vi "ProyectoBioCuinique Alpha 3.0.vi"() -> ()   [LabVIEW 2021]
uses:
  <vilib>/Utility/NIReport.llb/Report Type.ctl
  <extravilib>/ChannelInstances/Tag-dbl/Read With Abort.vi
  <extravilib>/ChannelInstances/Tag-bool/Read With Abort.vi
  <extravilib>/ChannelInstances/Tag-bool/Write With Abort.vi
  <extravilib>/ChannelInstances/Tag-dbl/Write With Abort.vi
  <vilib>/Instr/_visa.llb/VISA Configure Serial Port (Instr).vi
  <vilib>/MakerHub/LINX/Public/Utilities/Open Serial.vi
  <extravilib>/ChannelInstances/Tag-dbl/Instantiate.vi
  <extravilib>/ChannelInstances/Tag-bool/Instantiate.vi
  <extravilib>/ChannelInstances/Tag-dbl/EndpointRead.vi
  <vilib>/addons/_office/excel.llb/Excel Easy Table (str).vi
  <extravilib>/ChannelInstances/Tag-bool/EndpointRead.vi
  <extravilib>/ChannelInstances/Tag-bool/Endpoint.vi
  <extravilib>/ChannelInstances/Tag-dbl/Endpoint.vi
  <vilib>/Utility/NIReport.llb/NI_report.lvclass
  <vilib>/LabVIEW Interface for Arduino/LabVIEW Interface for Arduino.lvlib
  <vilib>/MakerHub/LINX/LMH-LINX.lvlib
  <vilib>/Utility/NIReport.llb/NI_ReportGenerationCore.lvlib
  <vilib>/addons/_office/NI_ReportGenerationToolkit.lvlib
  <vilib>/Utility/NIReport.llb/Excel/NI_Excel.lvclass
  <vilib>/MakerHub/LINX/Public/Sensors/Distance/Ultrasonic/Ultrasonic.lvlib
  <extravilib>/ChannelInstances/Tag-bool.lvlib
  <extravilib>/ChannelInstances/Tag-dbl.lvlib
panel:
  in  "Serial Port":refnum<visa-resource-name>="N/A"
  in  "template (empty)":path
  in  "Pin Bomba 1":u8
  in  "Pin Valvula 1":u8
  in  "Pin Valvula 2":u8
  out "HUMEDAD 2":dbl
  in  "VISA resource name":refnum<visa-resource-name>
  out "TEMPERATURA":dbl
  out "HUMEDAD":dbl(knob) scale=0.0..255.0
  out "Centimeters":dbl
  out "Slide":dbl(slide) scale=0.0..500.0
  out "BOMBA (11)":bool
  in  "Boolean 4":bool
  out "VALVULA (6)":bool
  in  "Boolean":bool
  out "VALVULA (5)":bool
  in  "stop":bool
  in  "VISA resource":refnum<visa-resource-name>
  # "VÁLVULA 1"
  # "BOMBA DE AGUA"
  # "VÁLVULA 2"
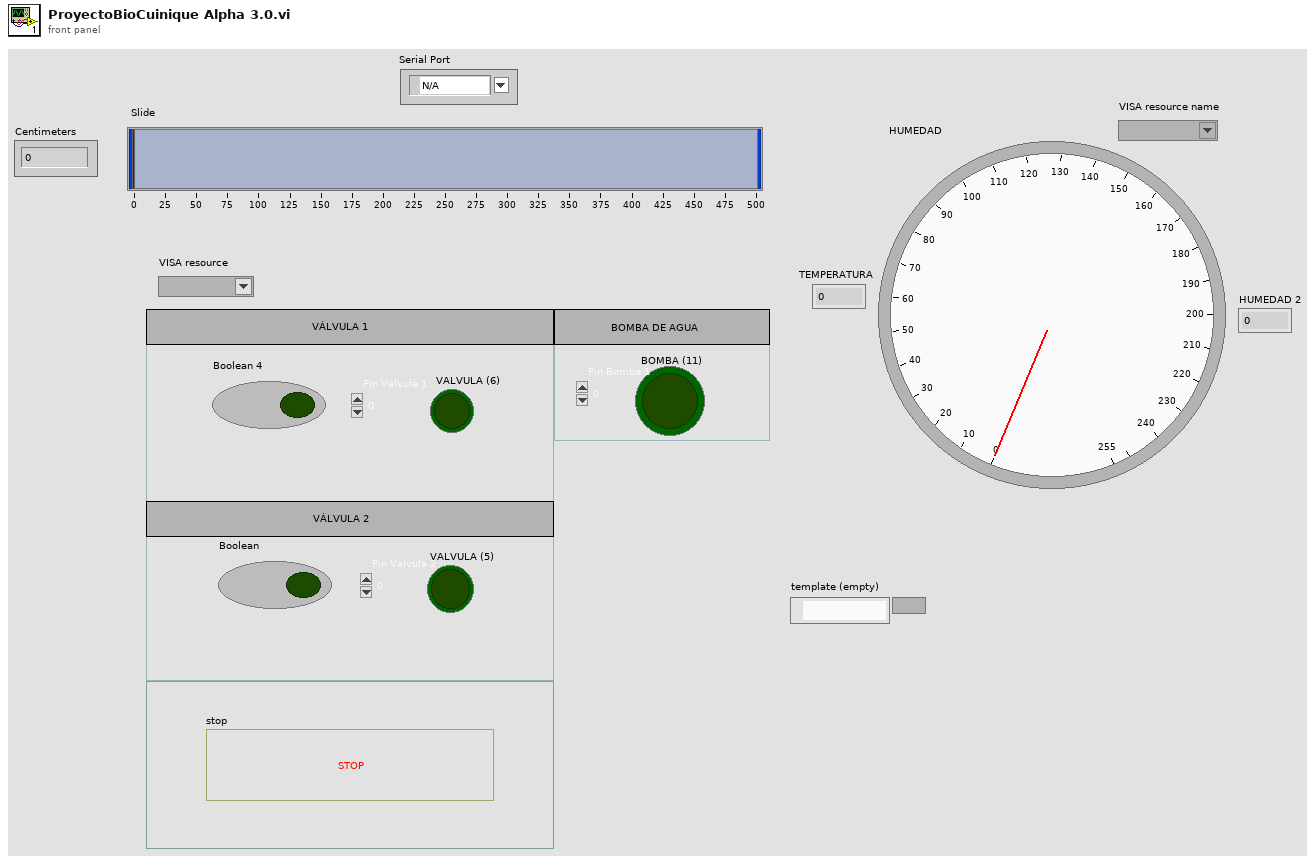
[diagram p1: front panel]
types:
  T1 = typedef "NI_ReportGenerationCore.lvlib/Report Type.ctl" = enum16{"HTML", "Word", "Excel"}
  T2 = typedef "LabVIEW Interface for Arduino.lvlib/Arduino Resource.ctl" = cluster{"VISA resource":refnum<visa-resource-name>, "Board Type":T3, "Connection Type":enum8{"USB / Serial"}, "Bytes Per Packet (15)":u8}
  T3 = typedef "LabVIEW Interface for Arduino.lvlib/Board Type.ctl" = enum16{"Uno", "Dimuelanove w/Atmega 328", "Mega 2560"}
  T4 = typedef "LMH-LINX.lvlib/LINX Ref.ctl" = cluster{"IO":T5, "Interface":T6, "LINX Device Config":T7}
  T5 = typedef "LMH-LINX.lvlib/Platform.ctl" = enum16{"Remote", "Local"}
  T6 = typedef "LMH-LINX.lvlib/Interface.ctl" = enum16{"Serial", "TCP"}
  T7 = typedef "LMH-LINX.lvlib/Device.lvlib/LINX Device Config.ctl" = cluster{"Interface":T6, "COM Port":refnum<visa-resource-name>, "TCP Configuration":T8, "Device Family":u8, "Device ID":u8, "Device Name":string, "TCP Ref":refnum<k5>, "Channels":T9}
  T8 = typedef "LMH-LINX.lvlib/Device.lvlib/TCP Config.ctl" = cluster{"IP Address":string, "Port":u16}
  T9 = typedef "LMH-LINX.lvlib/Channels.ctl" = cluster{"DI":u8[], "DO":u8[], "AI":u8[], "AO":u8[], "PWM":u8[], "QE":u8[], "UART":u8[], "I2C 2":u8[], "SPI":u8[], "CAN":u8[], "Servo":u8[], "AI Ref (V)":dbl, "AI Resolution (Bits)":u8, "AO Ref (V)":dbl, "AO Resolution (Bits)":u8}
  T10 = typedef "Tag-dbl.lvlib/))Channel.ctl" = refnum<queue>
  T11 = typedef "Tag-bool.lvlib/))Channel.ctl" = refnum<queue>
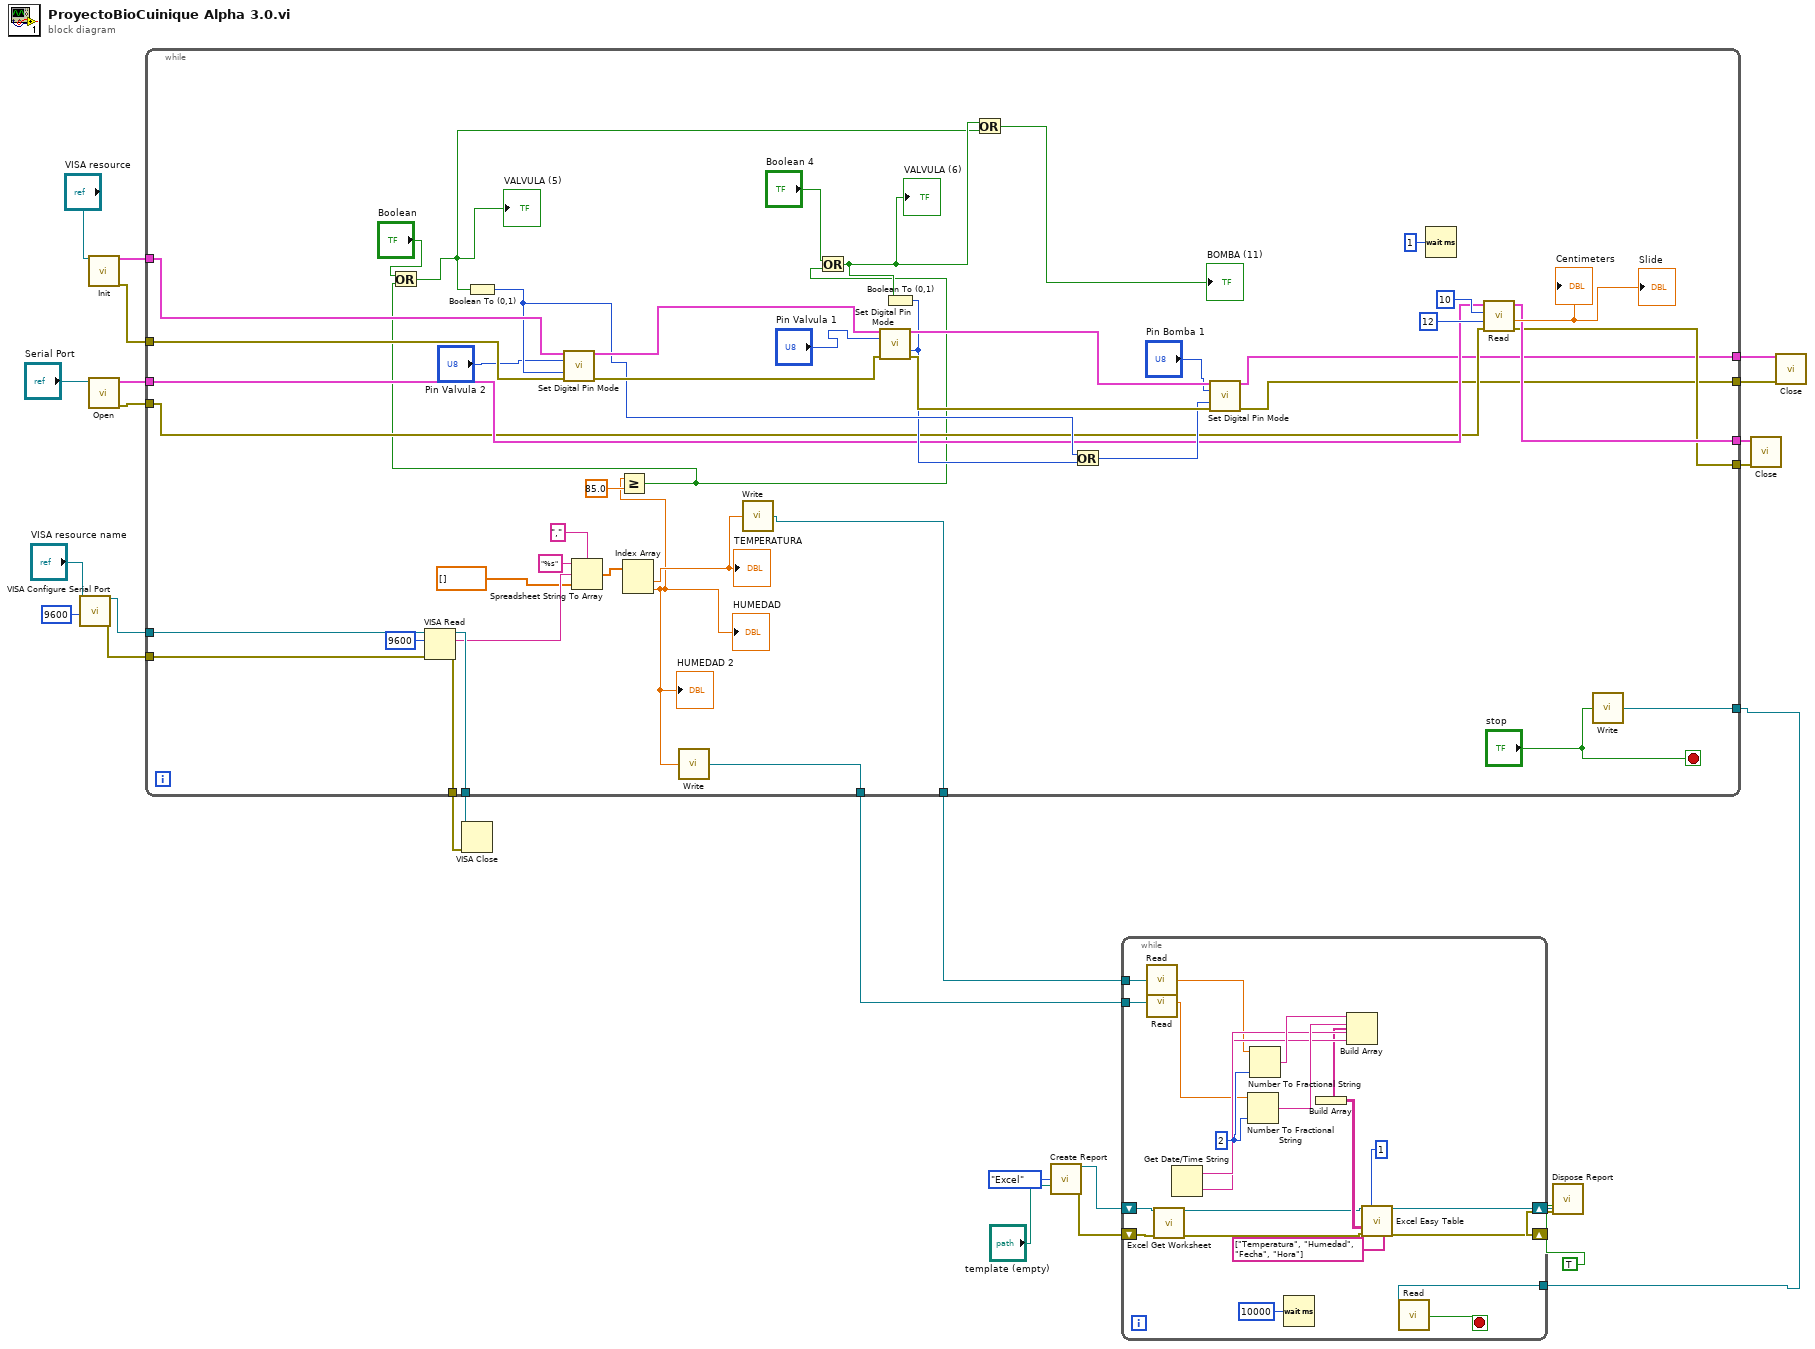
[diagram p0: block diagram]
diagram:
  n1 = call-poly "VISA Configure Serial Port"("VISA resource name"="VISA resource name", "baud rate (9600)"=u32 9600) -> ("VISA resource name out"=w17:refnum<visa-resource-name>, "error out"=w14:errorcluster)  [unwired: 12 in]
  n2 = call <vilib>:"Init.vi"("VISA resource"="VISA resource") -> ("Arduino Resource"=w25:T2, "error out"=w24:errorcluster)  [unwired: 17 in]
  n3 = call-poly <vilib>:"Open.vi"("Serial Port"="Serial Port") -> ("Error Out"=w23:errorcluster, "LINX Resource"=w22:T4)  [unwired: 8 in, 1 out]
  n4 = while {
    tunnel: w25 -> [w71]
    tunnel: w24 -> [w70]
    tunnel: w23 -> [w56]
    tunnel: w22 -> [w57]
    tunnel: [w55] -> w21
    tunnel: [w54] -> w20
    tunnel: [w53] -> w19
    tunnel: [w52] -> w18
    tunnel: w17 -> [w51]
    tunnel: [w50] -> w16
    tunnel: [w49] -> w15
    tunnel: w14 -> [w48]
    tunnel: [w32] -> w4
    tunnel: [w31] -> w3
    tunnel: [w30] -> w2
    stop <- "stop" stop-if-true
    n5 = VISA Read(VISA resource name=w51, byte count=u32 9600, error in (no error)=w48) -> (VISA resource name out=w49:refnum<visa-resource-name>, read buffer=w47:string, error out=w50:errorcluster)  [unwired: 1 out]
    n6 = Spreadsheet String To Array(delimiter (Tab)=",", format string="%s", spreadsheet string=w47, array type (2D Dbl)=dbl[] []) -> (array=w43:dbl[])
    n7 = Index Array(array=w43) -> (element #1=w42:dbl, element #2=w39:dbl)  [unwired: 2 in]
    "HUMEDAD" <- w39
    "TEMPERATURA" <- w42
    "HUMEDAD 2" <- w39
    n8 = Greater Or Equal?(x=w39, y=85.0) -> (x >= y?=w29:bool)
    n9 = Or(x="Boolean", y=w29) -> (x .or. y?=w27:bool)
    "VALVULA (5)" <- w27
    n10 = Boolean To (0,1)(Boolean=w27) -> (0, 1=w65:i16)
    n11 = call <vilib>:"Set Digital Pin Mode.vi"("Arduino Resource"=w71, "Digital I/O Pin"="Pin Valvula 2", "Pin Mode (Input)"=w65, "error in"=w70) -> ("Arduino Resource"=w69:T2, "error out"=w68:errorcluster)  [unwired: 10 in]
    n12 = call <extravilib>:"Write.vi"("element"=w39) -> ("channel"=w30:T10)  [unwired: 1 out]
    n13 = call <extravilib>:"Write.vi"("element"=w42) -> ("channel"=w31:T10)  [unwired: 1 out]
    n14 = Or(x="Boolean 4", y=w29) -> (x .or. y?=w37:bool)
    "VALVULA (6)" <- w37
    n15 = Boolean To (0,1)(Boolean=w37) -> (0, 1=w64:i16)
    n16 = call <vilib>:"Set Digital Pin Mode.vi"("Arduino Resource"=w69, "Digital I/O Pin"="Pin Valvula 1", "Pin Mode (Input)"=w64, "error in"=w68) -> ("Arduino Resource"=w66:T2, "error out"=w67:errorcluster)  [unwired: 10 in]
    n17 = Or(x=w37, y=w27) -> (x .or. y?=→"BOMBA (11)":bool)
    n18 = Or(x=w65, y=w64) -> (x .or. y?=w63:i16)
    n19 = call <vilib>:"Set Digital Pin Mode.vi"("Arduino Resource"=w66, "Digital I/O Pin"="Pin Bomba 1", "Pin Mode (Input)"=w63, "error in"=w67) -> ("Arduino Resource"=w53:T2, "error out"=w52:errorcluster)  [unwired: 10 in]
    n20 = Wait (ms)(milliseconds to wait=u32 1) -> ()  [unwired: 1 out]
    n21 = call <vilib>:"Read.vi"("Error In"=w56, "DO Channel"=u8 12, "DI Channel"=u8 10, "LINX Resource"=w57) -> ("Error Out"=w54:errorcluster, "Centimeters"=→"Centimeters" →"Slide":dbl, "LINX Resource"=w55:T4)  [unwired: 4 in, 1 out]
    n22 = call <extravilib>:"Write.vi"("element"="stop") -> ("channel"=w32:T11)  [unwired: 1 out]
  }
  n23 = VISA Close(VISA resource name=w15, error in (no error)=w16) -> ()  [unwired: 1 out]
  n24 = call <vilib>:"Create Report.vi"("report type"=Report_Type."Excel", "template (empty)"="template (empty)") -> ("report out"=w8:refnum<class "NI_report.lvclass">, "error out"=w9:errorcluster)  [unwired: 12 in]
  n25 = while {
    shift-right: [w81] -> w6
    shift-left: w9 -> [w86]
    shift-right: [w82] -> w7
    shift-left: w8 -> [w84]
    tunnel: w4 -> [w77]
    tunnel: w3 -> [w75]
    tunnel: w2 -> [w73]
    stop <- w76 stop-if-true
    w93 = i16 2 ("precision (6)")
    n26 = call <vilib>:"Read.vi"("channel"=w75) -> ("element"=w74:dbl)  [unwired: 1 in, 1 out]
    n27 = call <vilib>:"Read.vi"("channel"=w73) -> ("element"=w72:dbl)  [unwired: 1 in, 1 out]
    n28 = call <vilib>:"Excel Get Worksheet.vi"("report in"=w84, "error in (no error)"=w86) -> ("report out"=w83:refnum<class "NI_report.lvclass">, "error out"=w85:errorcluster)  [unwired: 12 in]
    n29 = Get Date/Time String() -> (date string=w90:string, time string=w89:string)  [unwired: 3 in]
    n30 = Number To Fractional String(number=w72, precision (6)=w93) -> (F-format string=w91:string)  [unwired: 2 in]
    n31 = Number To Fractional String(number=w74, precision (6)=w93) -> (F-format string=w92:string)  [unwired: 2 in]
    n32 = Wait (ms)(milliseconds to wait=u32 10000) -> ()  [unwired: 1 out]
    n33 = Build Array(w92, w91, w90, w89) -> (w88:string[])
    n34 = Build Array(w88) -> (w87:string[][])
    n35 = call-poly <vilib>:"Excel Easy Table.vi"("report in"=w83, "iteration"=1, "text data"=w87, "error in (no error)"=w85, "column headers"=string[] ["Temperatura", "Humedad", "Fecha", "Hora"]) -> ("report out"=w82:refnum<class "NI_report.lvclass">, "error out"=w81:errorcluster)  [unwired: 6 in, 3 out]
    n36 = call <vilib>:"Read.vi"("channel"=w77) -> ("element"=w76:bool)  [unwired: 1 in, 1 out]
  }
  n37 = call-dynamic "Dispose Report.vi"("report in"=w7, "save changes? (F)"=TRUE, "error in (no error)"=w6) -> ()  [unwired: 12 in, 1 out]
  n38 = call <vilib>:"Close.vi"("Error In"=w20, "LINX Resource"=w21) -> ()  [unwired: 9 in, 1 out]
  n39 = call <vilib>:"Close.vi"("Arduino Resource"=w19, "error in"=w18) -> ()  [unwired: 13 in, 1 out]
